vi "ECOG-Initialize Spectrogram.vi"(0 "params":T2, 7 "Map Ref":refnum<vi>, 11 "error in (no error)":errorcluster) -> (4 "params thru":T2, 13 "spectrogram":T1, 15 "error out":errorcluster)   [LabVIEW 2020]
uses:
  Typedefs/ECOG-Parameters.ctl
  Typedefs/ECOG-Spectrogram.ctl
  cce4edbd-d0dd-4855-81f2-beea96a88323.vi
  c4f31a37-5e52-4573-9ba0-0ad122ca2cdd.vi
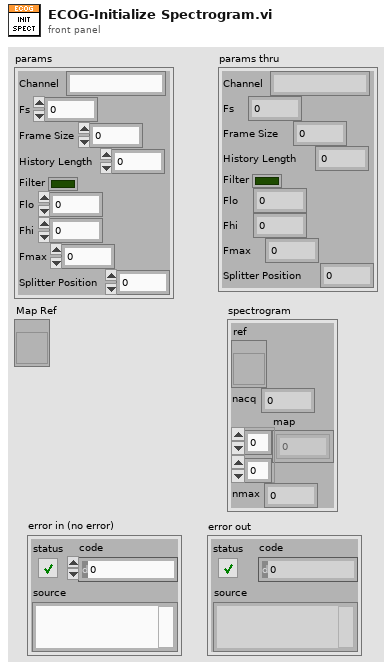
[diagram p1: front panel]
types:
  T1 = typedef "ECOG-Spectrogram.ctl" = cluster{"ref":refnum<vi>, "nacq":i32, "map":dbl[][], "nmax":i32}
  T2 = typedef "ECOG-Parameters.ctl" = cluster{"Channel":string, "Fs":dbl, "Frame Size":dbl, "History Length":dbl, "Filter":bool, "Flo":dbl, "Fhi":dbl, "Fmax":dbl, "Splitter Position":i32}
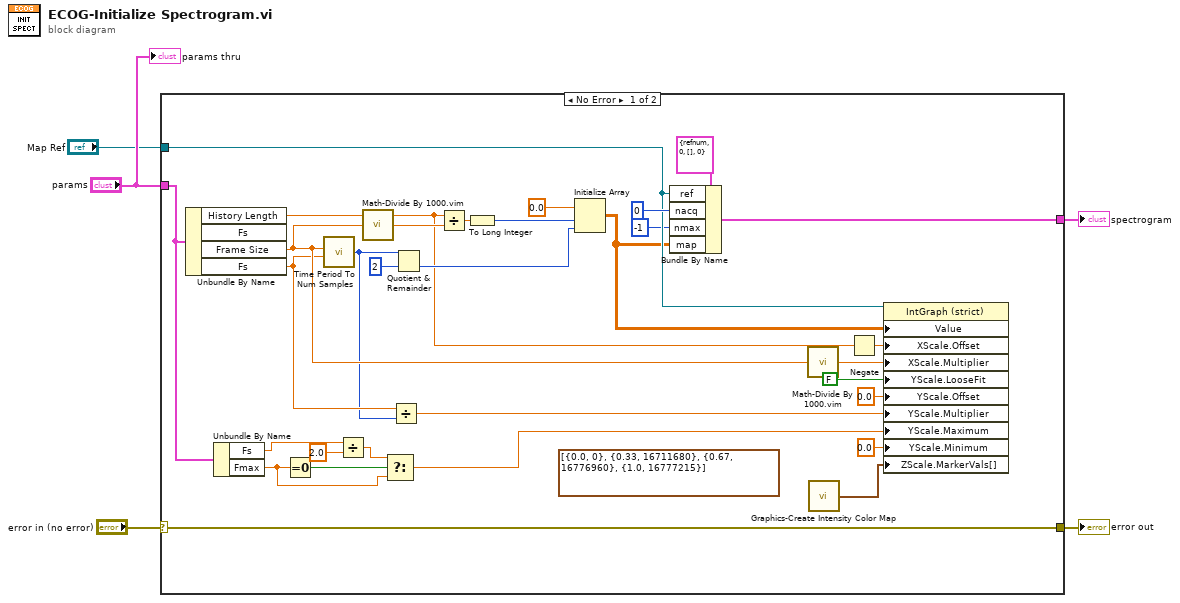
[diagram p0: block diagram]
diagram:
  n1 = case shown="No Error" "error in (no error)" {
    selector: "error in (no error)" -> [w35 w37]
    tunnel: "params" -> [w14 _]
    tunnel: [w35 w37] -> w4
    tunnel: "Map Ref" -> [w25 _]
    tunnel: [w36 _] -> w1
    frame No Error {
      (unwired) cluster{dbl, u32}[] [{0.0, 0}, {0.33, 16711680}, {0.67, 16776960}, {1.0, 16777215}] ("Z Scale.Marker Values[]")
      n2 = Unbundle By Name(w14) -> ("History Length"=w17:dbl, "Frame Size"=w23:dbl, "Fs"=w21:dbl)  [unwired: 1 out]
      n3 = Unbundle By Name(w14) -> ("Fs"=w9:dbl, "Fmax"=w12:dbl)
      n4 = Equal To 0?(x=w12) -> (x = 0?=w13:bool)
      n5 = call "Time Period To Num Samples.vi"("Duration (ms)"=w23, "Sampling rate (Hz)"=w21) -> ("Samples"=w20:i32)  [unwired: 5 in]
      n6 = Divide(x=w9, y=2.0) -> (x/y=w8:dbl)
      n7 = call "Math-Divide By 1000.vim"("X"=w23) -> ("1000X"=w29:dbl)
      n8 = Select(t=w8, s=w13, f=w12) -> (s? t:f=w11:dbl)
      n9 = Divide(x=w21, y=w20) -> (x/y=w19:dbl)
      n10 = Quotient & Remainder(x=w20, y=2) -> (floor(x/y)=w27:i32)  [unwired: 1 out]
      n11 = Divide(x=w17, y=w29) -> (x/y=w31:dbl)
      n12 = To Long Integer(number=w31) -> (32bit integer=w28:i32)
      n13 = Initialize Array(0.0, w28, w27) -> (w24:dbl[][])
      n14 = Bundle By Name(cluster=T1 {"ref"=refnum, "nacq"=0, "map"=[], "nmax"=0} ("spectrogram"), "ref"=w25, "nacq"=0, "nmax"=-1, "map"=w24) -> (w36:T1)
      n15 = call "Math-Divide By 1000.vim"("X"=w23) -> ("1000X"=w16:dbl)
      n16 = call "Graphics-Create Intensity Color Map.vi"() -> ("Array"=w6:cluster{dbl, "Color":u32}[])  [unwired: 1 in]
      n17 = Negate(x=w17) -> (-x=w18:dbl)
      n18 = property class="IntGraph (strict)"(reference=w25, "Value"=w24, "XScale.Offset"=w18, "XScale.Multiplier"=w16, "YScale.LooseFit"=FALSE ("Y Scale.Loose Fit"), "YScale.Offset"=0.0 ("Y Scale.Offset and Multiplier:Offset"), "YScale.Multiplier"=w19, "YScale.Maximum"=w11, "YScale.Minimum"=0.0 ("Y Scale.Range:Minimum"), "ZScale.MarkerVals[]"=w6) -> ()  [unwired: 1 in, 2 out]
    }
    frame Error {
    }
  }
  "error out" <- w4
  "spectrogram" <- w1
  "params thru" <- "params"
